vi "TCP聊天 passive.vi"() -> ()   [LabVIEW 2011]
doc: "说明显示的交互式发送和接收信息对话框可用于TCP连接间的通信。将在指定端口监听10秒钟。如未检测到任何连接，监听将超时。如检测到连接，将等待用户在“输入行”字符串输入控件中输入数据。单击回车键后，所输字符串将发送至端口并传递至TCP Communicator - Active.vi中显示的字符串控件中。\n\nTCP Communicator - Active.vi和TCP Communicator - Passive.vi的主要区别是主动VI将建立一个连接，而被动VI将等待该连接。\n\n<B>注：</B>需要TCP Communicator - Active.vi。"
panel:
  in  "Machine":string="localhost" caption="IP"
  in  "Port":u16=6342 caption="端口"
  out "Their Response:":string caption="对方的话:"
  in  "stop":bool caption="停止"
  out "You Typed:":string caption="我说的话:"
  in  "Input Line":string caption="输入"
  # "基于TCP/IP的简易聊天程序"
  # "步骤:\n1. 打开TCP\n    Communicator - Active.vi。\n2. 运行本VI。\n3. 运行TCP Communicator - \n    Active.vi。\n4.在输入行\n    字符串控件中输入\n    并单击回车。\n5. 在其它VI的输入行\n    中输入并单击\n    回车。\n6. 按停止按钮可结束该操作。"
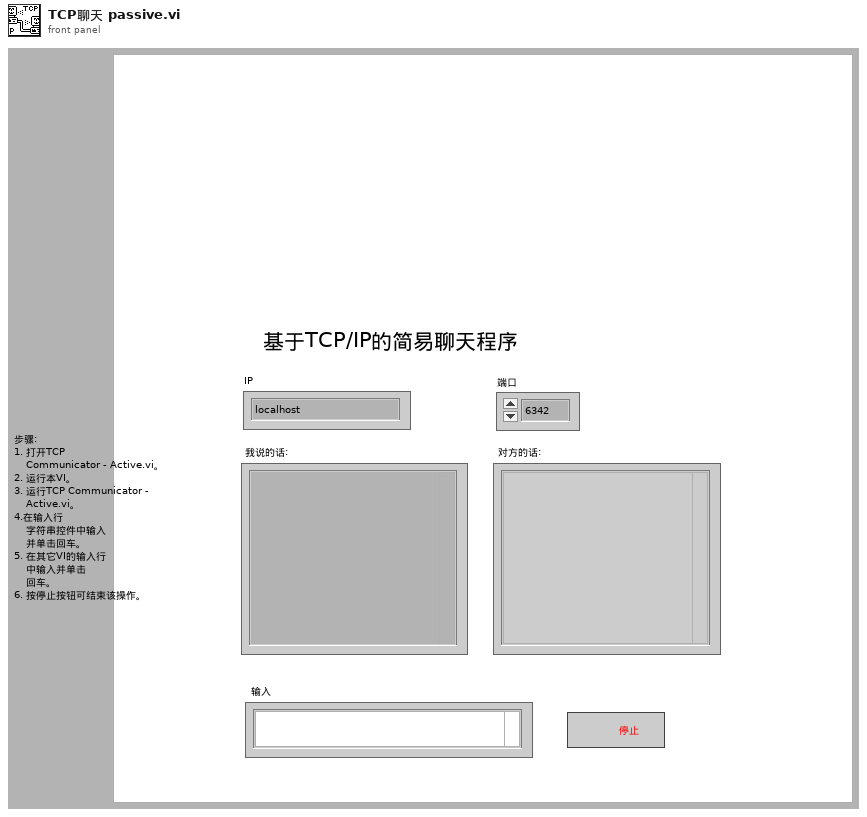
[diagram p1: front panel]
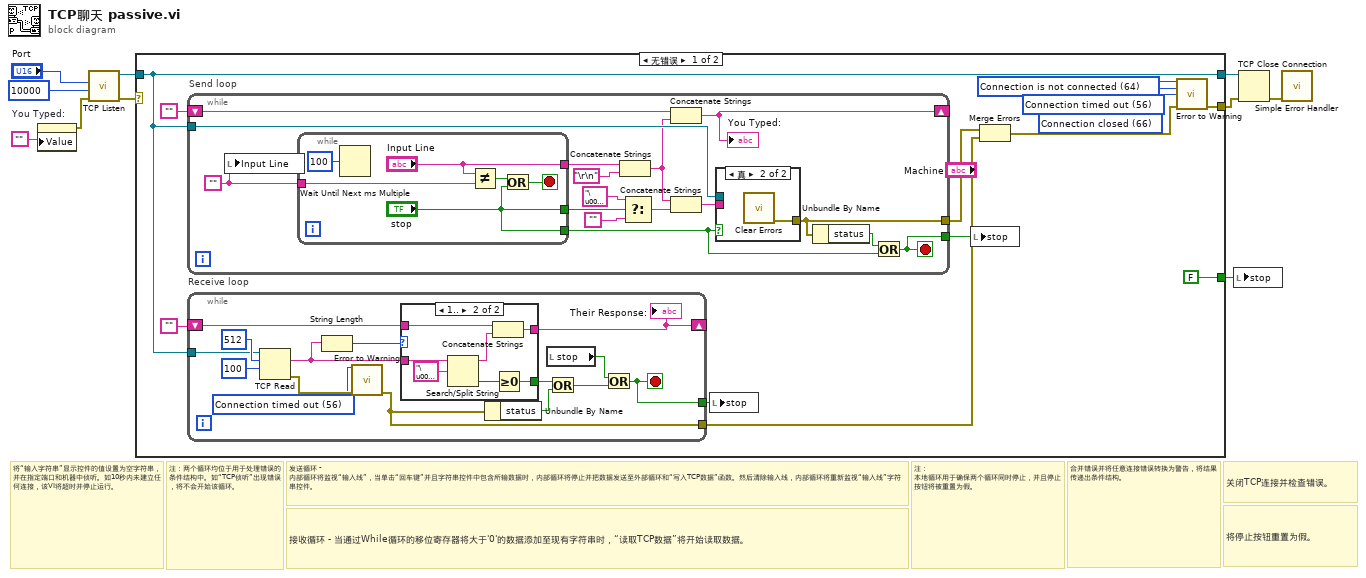
[diagram p0: block diagram]
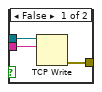
[diagram p2: hidden frame]
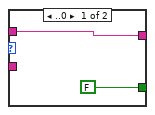
[diagram p3: hidden frame]
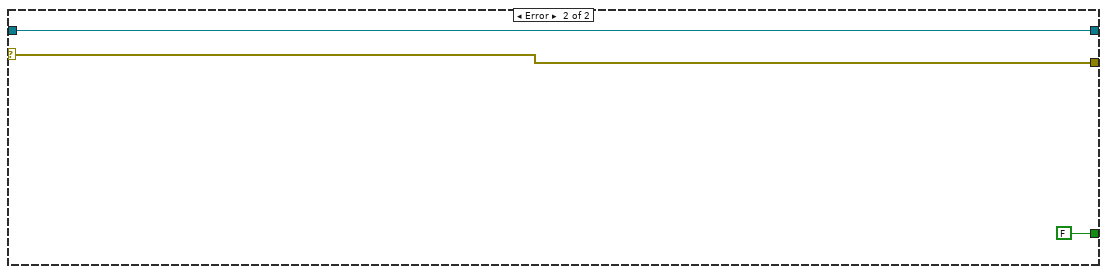
[diagram p4: hidden frame]
diagram:
  # "将停止按钮重置为假。"
  # "关闭TCP连接并检查错误。"
  # "注：两个循环均位于用于处理错误的条件结构中。如“TCP侦听”出现错误，将不会开始该循环。"
  # "合并错误并将任意连接错误转换为警告，将结果传递出条件结构。"
  # "注： 本地循环用于确保两个循环同时停止，并且停止按钮将被重置为假。"
  # "接收循环 - 当通过While循环的移位寄存器将大于'0'的数据添加至现有字符串时，“读取TCP数据”将开始读取数据。"
  # "发送循环 - 内部循环将监视“输入线”，当单击“回车键”并且字符串控件中包含所输数据时，内部循环将停止并把数据发送至外部循环和“写入TCP数据”函数。然后清除输入线，内部循环将重新监视“输入线”字符串控件。"
  # "将“输入字符串”显示控件的值设置为空字符串，并在指定端口和机器中侦听。如10秒内未建立任何连接，该VI将超时并停止运行。"
  n1 = property on="You Typed:" class="Str"("Value"="") -> (error out=w4:errorcluster)  [unwired: 2 in, 1 out]
  n2 = call <vilib>:"TCP Listen.vi"("error in (no error)"=w4, "timeout ms (wait forever: -1)"=10000, "port"="Port") -> ("error out"=w5:errorcluster, "connection ID"=w6:refnum<k5>)  [unwired: 4 in, 3 out]
  n3 = case shown="无错误" w5 {
    selector: w5 -> [_ w75]
    tunnel: [w15 w75] -> w8
    tunnel: w6 -> [w21 w76]
    tunnel: [w21 w76] -> w9
    tunnel: [FALSE FALSE] -> w1
    frame No Error {
      w12 = 56 items=["No Error", "Argument Error", "Memory Full", "Out of Zone", "End of File", "File Already Open", "Generic File IO Error", "File Not Found", "File Permission Error", "Disk Full", "Duplicate Path", "Too Many Files Open", "Not Enabled", "Resource File Not Found", "Cannot Add Resource", "Resource Not Found", "Image Not Found", "Image Memory Error", "Pen Does Not Exist", "Config Bad Type", "Config Token Not Found", "Config Parse Error", "Config Memory Error", "Bad External Code Format", "Bad External Code Offset", "External Code Not Present", "Null Window", "Destroy Window Mixup", "Null Menu", "Print Aborted", "Bad Print Record", "Print Driver Error", "Windows Error During Print", "Memory Error During Print", "Print Dialog Error", "Generic Print Error", "Invalid Device Refnum", "Device Not Found", "Device Parameter Error", "Device Unit Error", "Can't Open Device", "Device Call Aborted", "Generic Error", "Cancelled By User", "Object ID Too Low", "Object ID Too High", "Object Not In Heap", "Unknown Heap", "Bad DefProc ID", "DefProc Not In Table", "Message Out Of Range", "Null Method", "Unknown Message", "Manager Call Not Supported", "Bad address", "Connection In progress", "Connection timed out", "Connection is already in progress", "Network attribute not supported", "Network error", "Address in use", "System out of memory", "Connection aborted", "Connection refused", "Connection is not connected", "Connection is already connected", "Connection closed", "Initialize error (interapplication manager)", "Bad occurrence", "Wait on unbound occurrence handler", "Occurrence queue overflow", "Bad path", "Semaphore not signaled", "Unrecognized type (interapplication manager)"] ("2nd Error to Convert")
      w16 = 66 items=["No Error", "Argument Error", "Memory Full", "Out of Zone", "End of File", "File Already Open", "Generic File IO Error", "File Not Found", "File Permission Error", "Disk Full", "Duplicate Path", "Too Many Files Open", "Not Enabled", "Resource File Not Found", "Cannot Add Resource", "Resource Not Found", "Image Not Found", "Image Memory Error", "Pen Does Not Exist", "Config Bad Type", "Config Token Not Found", "Config Parse Error", "Config Memory Error", "Bad External Code Format", "Bad External Code Offset", "External Code Not Present", "Null Window", "Destroy Window Mixup", "Null Menu", "Print Aborted", "Bad Print Record", "Print Driver Error", "Windows Error During Print", "Memory Error During Print", "Print Dialog Error", "Generic Print Error", "Invalid Device Refnum", "Device Not Found", "Device Parameter Error", "Device Unit Error", "Can't Open Device", "Device Call Aborted", "Generic Error", "Cancelled By User", "Object ID Too Low", "Object ID Too High", "Object Not In Heap", "Unknown Heap", "Bad DefProc ID", "DefProc Not In Table", "Message Out Of Range", "Null Method", "Unknown Message", "Manager Call Not Supported", "Bad address", "Connection In progress", "Connection timed out", "Connection is already in progress", "Network attribute not supported", "Network error", "Address in use", "System out of memory", "Connection aborted", "Connection refused", "Connection is not connected", "Connection is already connected", "Connection closed", "Initialize error (interapplication manager)", "Bad occurrence", "Wait on unbound occurrence handler", "Occurrence queue overflow", "Bad path", "Semaphore not signaled", "Unrecognized type (interapplication manager)"] ("3rd Error to Convert")
      w17 = 64 items=["No Error", "Argument Error", "Memory Full", "Out of Zone", "End of File", "File Already Open", "Generic File IO Error", "File Not Found", "File Permission Error", "Disk Full", "Duplicate Path", "Too Many Files Open", "Not Enabled", "Resource File Not Found", "Cannot Add Resource", "Resource Not Found", "Image Not Found", "Image Memory Error", "Pen Does Not Exist", "Config Bad Type", "Config Token Not Found", "Config Parse Error", "Config Memory Error", "Bad External Code Format", "Bad External Code Offset", "External Code Not Present", "Null Window", "Destroy Window Mixup", "Null Menu", "Print Aborted", "Bad Print Record", "Print Driver Error", "Windows Error During Print", "Memory Error During Print", "Print Dialog Error", "Generic Print Error", "Invalid Device Refnum", "Device Not Found", "Device Parameter Error", "Device Unit Error", "Can't Open Device", "Device Call Aborted", "Generic Error", "Cancelled By User", "Object ID Too Low", "Object ID Too High", "Object Not In Heap", "Unknown Heap", "Bad DefProc ID", "DefProc Not In Table", "Message Out Of Range", "Null Method", "Unknown Message", "Manager Call Not Supported", "Bad address", "Connection In progress", "Connection timed out", "Connection is already in progress", "Network attribute not supported", "Network error", "Address in use", "System out of memory", "Connection aborted", "Connection refused", "Connection is not connected", "Connection is already connected", "Connection closed", "Initialize error (interapplication manager)", "Bad occurrence", "Wait on unbound occurrence handler", "Occurrence queue overflow", "Bad path", "Semaphore not signaled", "Unrecognized type (interapplication manager)"] ("1st Error to Convert")
      n4 = while "Send loop" {
        tunnel: w21 -> [w36]
        tunnel: [w38] -> w13
        tunnel: [w27] -> w19
        shift-left: "" -> [w39]
        shift-right: [w37] -> _
        stop <- w38 stop-if-true
        w25 = ""
        n5 = local write "Input Line"(w25) -> ()
        n6 = while {
          tunnel: ["stop"] -> w32
          tunnel: ["stop"] -> w24
          tunnel: ["Input Line"] -> w33
          tunnel: w25 -> [w41]
          stop <- w43 stop-if-true
          n7 = Wait Until Next ms Multiple(millisecond multiple=u32 100) -> ()  [unwired: 1 out]
          n8 = Not Equal?(x="Input Line", y=w41) -> (x != y?=w44:bool)
          n9 = Or(x=w44, y="stop") -> (x .or. y?=w43:bool)
        }
        n10 = Concatenate Strings(w33, "\r\n") -> (w29:string)
        n11 = Select(t="\u0004", s=w32, f="") -> (s? t:f=w34:string)
        n12 = Concatenate Strings(w39, w29) -> (w37:string)
        "You Typed:" <- w37
        n13 = Concatenate Strings(w29, w34) -> (w28:string)
        n14 = case shown="真" w24 {
          tunnel: w28 -> [w48 _]
          tunnel: [w47 w49] -> w27
          tunnel: w36 -> [w46 _]
          frame False {
            n15 = TCP Write(connection ID=w46, data in=w48) -> (error out=w47:errorcluster)  [unwired: 2 in, 2 out]
          }
          frame True {
            n16 = call <vilib>:"Clear Errors.vi"() -> ("error out"=w49:errorcluster)  [unwired: 7 in]
          }
        }
        n17 = Unbundle By Name(w27) -> ("status"=w26:bool)
        n18 = Or(x=w26, y=w24) -> (x .or. y?=w38:bool)
      }
      n19 = while "Receive loop" {
        shift-left: "" -> [w60]
        shift-right: [w59] -> _
        tunnel: [w61] -> w14
        tunnel: [w53] -> w20
        tunnel: w21 -> [w62]
        stop <- w61 stop-if-true
        w54 = 56 items=["No Error", "Argument Error", "Memory Full", "Out of Zone", "End of File", "File Already Open", "Generic File IO Error", "File Not Found", "File Permission Error", "Disk Full", "Duplicate Path", "Too Many Files Open", "Not Enabled", "Resource File Not Found", "Cannot Add Resource", "Resource Not Found", "Image Not Found", "Image Memory Error", "Pen Does Not Exist", "Config Bad Type", "Config Token Not Found", "Config Parse Error", "Config Memory Error", "Bad External Code Format", "Bad External Code Offset", "External Code Not Present", "Null Window", "Destroy Window Mixup", "Null Menu", "Print Aborted", "Bad Print Record", "Print Driver Error", "Windows Error During Print", "Memory Error During Print", "Print Dialog Error", "Generic Print Error", "Invalid Device Refnum", "Device Not Found", "Device Parameter Error", "Device Unit Error", "Can't Open Device", "Device Call Aborted", "Generic Error", "Cancelled By User", "Object ID Too Low", "Object ID Too High", "Object Not In Heap", "Unknown Heap", "Bad DefProc ID", "DefProc Not In Table", "Message Out Of Range", "Null Method", "Unknown Message", "Manager Call Not Supported", "Bad address", "Connection In progress", "Connection timed out", "Connection is already in progress", "Network attribute not supported", "Network error", "Address in use", "System out of memory", "Connection aborted", "Connection refused", "Connection is not connected", "Connection is already connected", "Connection closed", "Initialize error (interapplication manager)", "Bad occurrence", "Wait on unbound occurrence handler", "Occurrence queue overflow", "Bad path", "Semaphore not signaled", "Unrecognized type (interapplication manager)"] ("1st Error to Convert")
        n20 = TCP Read(connection ID=w62, bytes to read=512, 9:100) -> (data out=w58:string, error out=w55:errorcluster)  [unwired: 2 in, 1 out]
        n21 = String Length(string=w58) -> (length=w64:i32)
        n22 = call <vilib>:"Error to Warning.vi"("1st Error to Convert"=w54, "error in"=w55) -> ("warning out"=w53:errorcluster)  [unwired: 13 in]
        n23 = case shown="1.." w64 {
          tunnel: w58 -> [_ w70]
          tunnel: w60 -> [w66 w73]
          tunnel: [w66 w72] -> w59
          tunnel: [FALSE w67] -> w57
          frame ..0 {
          }
          frame 1.. {
            n24 = Search/Split String(string=w70, search string/char (-)="\u0004") -> (substring before match=w69:string, offset of match=w68:i32)  [unwired: 1 in, 1 out]
            n25 = Concatenate Strings(w73, w69) -> (w72:string)
            n26 = Greater Or Equal To 0?(x=w68) -> (x >= 0?=w67:bool)
          }
        }
        "Their Response:" <- w59
        n27 = Unbundle By Name(w53) -> ("status"=w52:bool)
        n28 = local read "stop"() -> (w51:bool)
        n29 = Or(x=w57, y=w52) -> (x .or. y?=w50:bool)
        n30 = Or(x=w51, y=w50) -> (x .or. y?=w61:bool)
      }
      n31 = local write "stop"(w14) -> ()
      n32 = local write "stop"(w13) -> ()
      n33 = Merge Errors(w19, w20) -> (w18:errorcluster)
      n34 = call <vilib>:"Error to Warning.vi"("1st Error to Convert"=w17, "2nd Error to Convert"=w12, "3rd Error to Convert"=w16, "error in"=w18) -> ("warning out"=w15:errorcluster)  [unwired: 11 in]
    }
    frame Error {
    }
  }
  n35 = local write "stop"(w1) -> ()
  n36 = TCP Close Connection(connection ID=w9, error in (no error)=w8) -> (error out=w7:errorcluster)  [unwired: 1 in, 1 out]
  n37 = call <vilib>:"Simple Error Handler.vi"("error in (no error)"=w7) -> ()  [unwired: 4 in, 5 out]
